vi "Configure Decibel.vi"(8 "error in (no error)":errorcluster, 9 "dB Reference Value (0: Unity)":i32(ring) items=["Unity", "R50", "R75", "R600"], 10 "Enable dB (T: ON)":bool=TRUE, 11 "VISA resource name":refnum<visa-resource-name>) -> (0 "error out":errorcluster, 3 "VISA resource name out":refnum<visa-resource-name>)   [LabVIEW 2011, in "Fluke 8508.lvlib"]
doc: "This VI sets the decibel function on the instrument and configures the dB reference value.\n\nCombinations of math VIs are allowed, but they must be performed in the following order:\n1. Averaging\n2. Multiplication \n3. Subtraction \n4. Division\n5. Decibels"
uses:
  Fluke 8508.lvlib
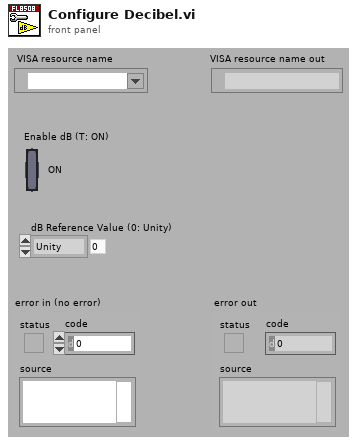
[diagram p1: front panel]
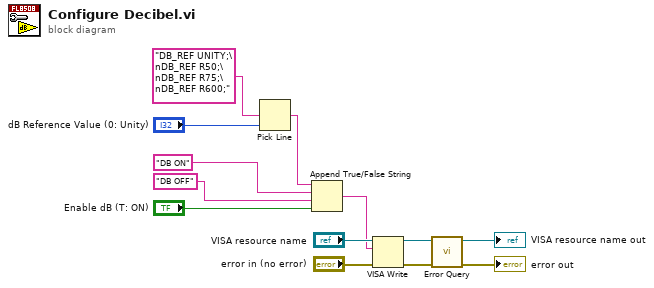
[diagram p0: block diagram]
diagram:
  n1 = Pick Line(multi-line string="DB_REF UNITY;\nDB_REF R50;\nDB_REF R75;\nDB_REF R600;" ("format string"), line index="dB Reference Value (0: Unity)") -> (output string=w9:string)  [unwired: 1 in]
  n2 = Append True/False String(1:"Enable dB (T: ON)", 2:"DB OFF" ("true string"), 3:"DB ON" ("true string"), 4:w9) -> (0:w6:string)
  n3 = VISA Write(VISA resource name="VISA resource name", write buffer=w6, error in (no error)="error in (no error)") -> (VISA resource name out=w2:refnum<visa-resource-name>, error out=w4:errorcluster)  [unwired: 1 out]
  n4 = call "Error Query.vi"("error in (no error)"=w4, "VISA resource name"=w2) -> ("error out"=→"error out":errorcluster, "VISA resource name out"=→"VISA resource name out":refnum<visa-resource-name>)  [unwired: 6 in, 2 out]
